vi "子面板测试.vi"() -> ()   [LabVIEW 2018]
panel:
  in  "停止":bool
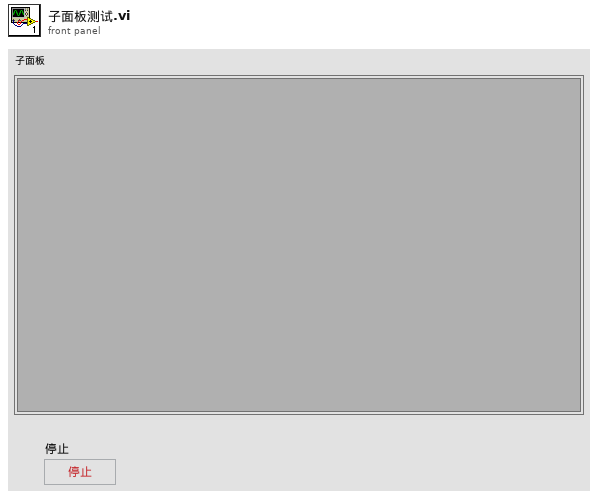
[diagram p1: front panel]
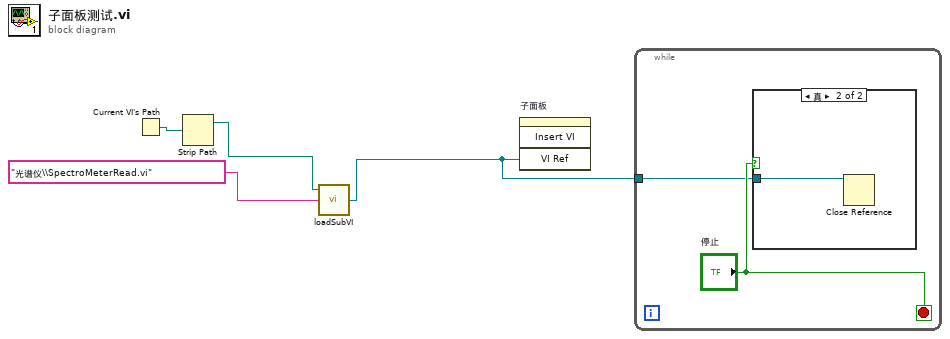
[diagram p0: block diagram]
diagram:
  n1 = Current VI's Path() -> (path=w4:path)
  n2 = Strip Path(path=w4) -> (stripped path=w3:path)  [unwired: 1 out]
  n3 = call "loadSubVI.vi"("VI名称"="光谱仪\\SpectroMeterRead.vi" ("名称或相对路径"), "基路径"=w3) -> ("SubVIRef"=w1:refnum<vi>)  [unwired: 2 in, 1 out]
  n4 = invoke on="子面板" class="SubPnl" method="Insert VI"("VI Ref"=w1) -> ()  [unwired: 3 in, 4 out]
  n5 = while {
    tunnel: w1 -> [w5]
    stop <- "停止" stop-if-true
    n6 = case shown="真" "停止" {
      tunnel: w5 -> [_ w7]
      frame False {
      }
      frame True {
        n7 = Close Reference(reference=w7) -> ()  [unwired: 1 in, 1 out]
      }
    }
  }
